vi "Universal NT Variable Writer.vi"() -> ()   [LabVIEW 2015]
uses:
  <vilib>/Rock Robotics/Network Tables/NT Write Boolean.vi
  <vilib>/Rock Robotics/Network Tables/NT Write Number.vi
  <vilib>/Rock Robotics/Network Tables/NT Write String.vi
  <vilib>/Rock Robotics/Network Tables/NT Write Boolean Array.vi
  <vilib>/Rock Robotics/Network Tables/NT Write Numeric Array.vi
  <vilib>/Rock Robotics/Network Tables/NT Write String Array.vi
panel:
  out "Tree":string(tree)
  out "Connected":bool
  out "Connection Count":i32
  out "Bind Failures":i32
  out "error out":errorcluster
  in  "Write":bool
  in  "Variable Value Selector":T1(tab)
  in  "Boolean":bool
  in  "Number":dbl
  in  "String":string
  in  "Boolean Array":bool[](array[boolean])
  in  "Numeric Array":dbl[](array[numeric])
  in  "String Array":string[](array[string])
  in  "Variable":string
  in  "stop":bool
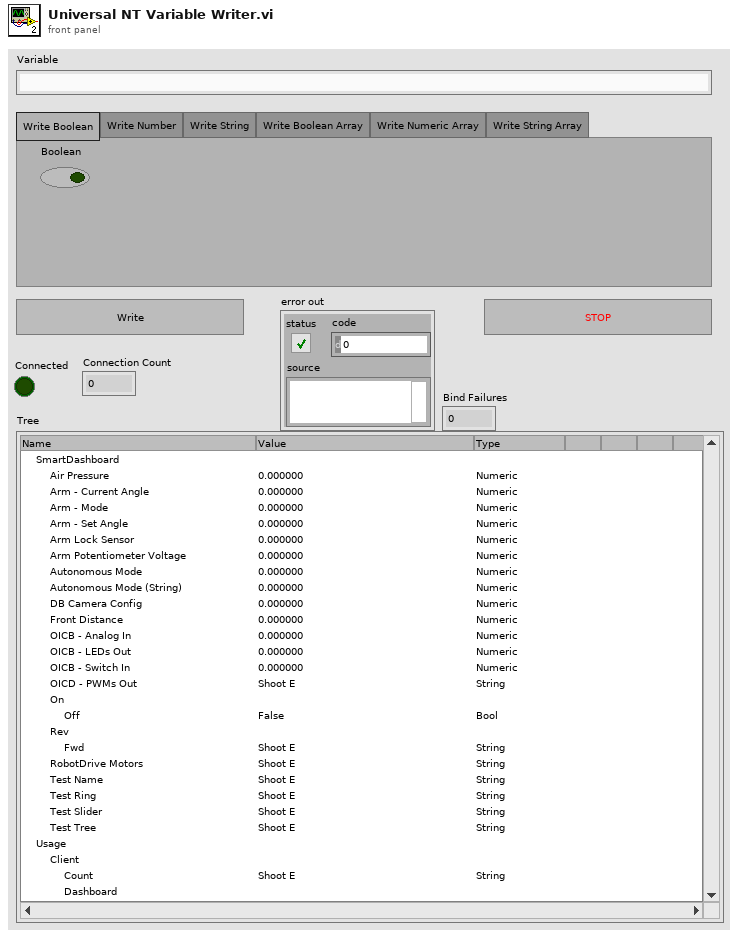
[diagram p1: front panel]
types:
  T1 = enum32{"Write Boolean", "Write Number", "Write String", "Write Boolean Array", "Write Numeric Array", "Write String Array"}
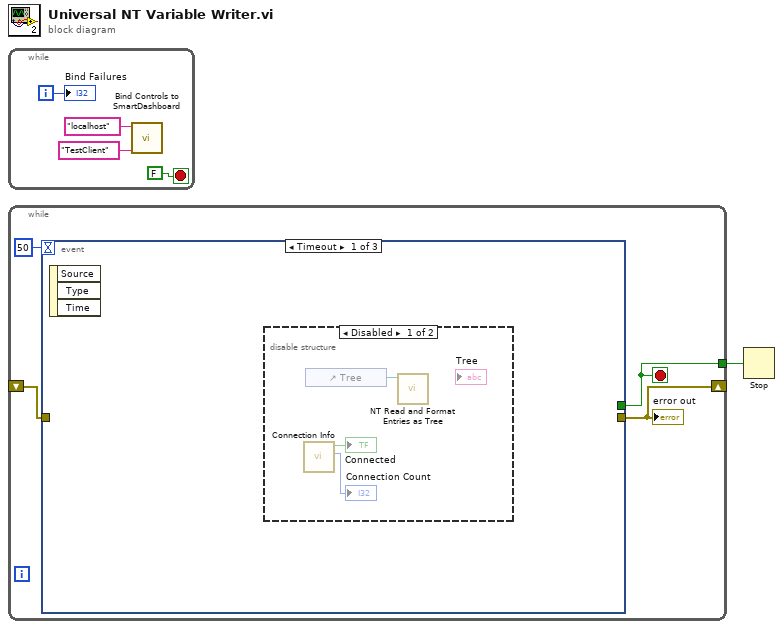
[diagram p0: block diagram]
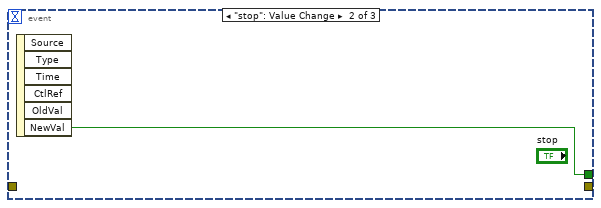
[diagram p3: hidden frame]
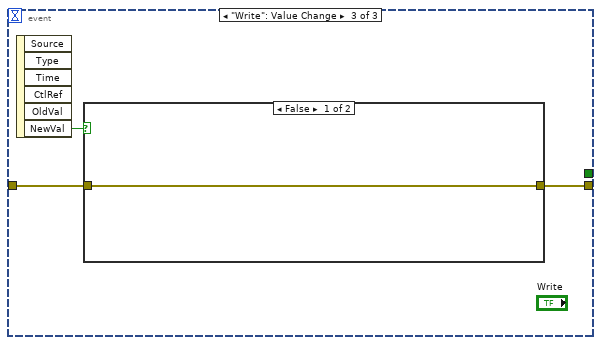
[diagram p4: hidden frame]
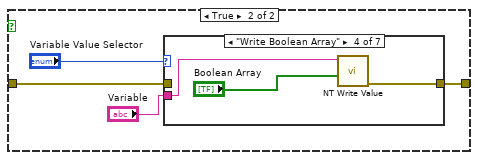
[diagram p5: hidden frame]
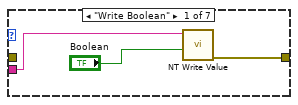
[diagram p6: hidden frame]
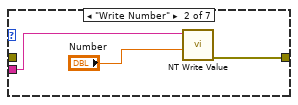
[diagram p7: hidden frame]
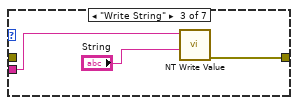
[diagram p8: hidden frame]
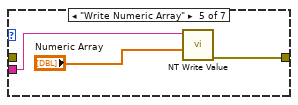
[diagram p9: hidden frame]
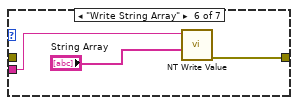
[diagram p10: hidden frame]
diagram:
  n1 = while {
    i -> [w2]
    stop <- FALSE stop-if-true
    n2 = call <vilib>:"Bind Controls to SmartDashboard.vi"("Client Name"="TestClient", "Server IP Address"="localhost") -> ()  [unwired: 10 in]
    "Bind Failures" <- w2
  }
  n3 = while {
    tunnel: [w9] -> w1
    shift-right: [w8] -> _
    shift-left: _ -> [w7]
    stop <- w9 stop-if-true
    n4 = event shown="[0] Timeout" {
      selector: _ -> [_ _ _]
      dyn-events: _ -> [_ _ _]
      timeout: 50 -> [_ _ _]
      tunnel: [_ w13 _] -> w9
      tunnel: [_ _ w15] -> w8
      tunnel: w7 -> [_ _ w14]
      event Timeout {
        n5 = event-data() -> ()  [unwired: 1 in, 3 out]
        n6 = disable-structure shown="Disabled" {
          frame Disabled {
            n7 = call <vilib>:"Connection Info.vi"() -> ("Connection Count"=→"Connection Count":i32, "Connected"=→"Connected":bool)  [unwired: 10 in]
            n8 = control-ref of="Tree"() -> (w12:refnum<vi>)
            n9 = call <vilib>:"NT Read and Format Entries as Tree.vi"("Tree Refnum"=w12) -> ()  [unwired: 9 in, 2 out]
          }
          frame Enabled {
          }
        }
      }
      event "stop": Value Change {
        n10 = event-data() -> ("NewVal"=w13:bool)  [unwired: 1 in, 5 out]
      }
      event "Write": Value Change {
        n11 = event-data() -> ("NewVal"=w16:bool)  [unwired: 1 in, 5 out]
        n12 = case shown="False" w16 {
          tunnel: [w17 w19] -> w15
          tunnel: w14 -> [w17 w18]
          frame False {
          }
          frame True {
            n13 = case shown="\"Write Boolean Array\"" "Variable Value Selector" {
              tunnel: "Variable" -> [w24 w27 w30 w33 w36 w39 _]
              tunnel: [w22 w25 w28 w31 w34 w37 w40] -> w19
              tunnel: w18 -> [_ _ _ _ _ _ w40]
              frame "Write Boolean" {
                n14 = call-poly <vilib>:"NT Write Value.vi"("Boolean"="Boolean", "Name"=w24) -> ("error out"=w22:errorcluster)  [unwired: 9 in]
              }
              frame "Write Number" {
                n15 = call-poly <vilib>:"NT Write Value.vi"("Numeric"="Number", "Name"=w27) -> ("error out"=w25:errorcluster)  [unwired: 9 in]
              }
              frame "Write String" {
                n16 = call-poly <vilib>:"NT Write Value.vi"("String"="String", "Name"=w30) -> ("error out"=w28:errorcluster)  [unwired: 9 in]
              }
              frame "Write Boolean Array" {
                n17 = call-poly <vilib>:"NT Write Value.vi"("Boolean Array"="Boolean Array", "Name"=w33) -> ("error out"=w31:errorcluster)  [unwired: 9 in]
              }
              frame "Write Numeric Array" {
                n18 = call-poly <vilib>:"NT Write Value.vi"("Numeric Array"="Numeric Array", "Name"=w36) -> ("error out"=w34:errorcluster)  [unwired: 9 in]
              }
              frame "Write String Array" {
                n19 = call-poly <vilib>:"NT Write Value.vi"("String Array"="String Array", "Name"=w39) -> ("error out"=w37:errorcluster)  [unwired: 9 in]
              }
              frame Default {
              }
            }
          }
        }
      }
    }
    "error out" <- w8
  }
  n20 = Stop(stop? (T)=w1) -> ()
